vi "Example_USBCSwitch.vi"() -> ()   [LabVIEW 2021, in "BrainStem2_LabVIEW_Library.lvlib"]
uses:
  BrainStem2_LabVIEW_Library.lvlib
panel:
  out "Mux 3 Voltage":i32
  out "USB 0 CC1 Voltage":u32
  out "USB 0 CC1 Current":i32
  out "USB 0 CC2 Voltage":i32
  out "USB 0 CC1 Current":i32
  out "Mux 2 Voltage":i32
  out "USB 0 CC1 Voltage":i32
  out "USB 0 CC1 Current":i32
  out "USB 0 CC2 Voltage":i32
  out "USB 0 CC1 Current":i32
  out "Mux 1 Voltage":i32
  out "USB 0 CC1 Voltage":i32
  out "USB 0 CC1 Current":i32
  out "USB 0 CC2 Voltage":i32
  out "USB 0 CC1 Current":i32
  out "USB 0 CC2 Voltage":i32
  out "USB 0 CC1 Current":i32
  out "USB 0 CC1 Current":i32
  out "USB 0 CC1 Voltage":i32
  out "Mux 0 Voltage":i32
  out "USB 0 Voltage":i32
  out "USB 0 Current":i32
  out "USB 0 Voltage":i32
  out "USB 0 Current":i32
  out "USB 0 Voltage":i32
  out "USB 0 Current":i32
  out "USB 0 Voltage":i32
  out "USB 0 Current":i32
  # "Mux Channel 0 Values:"
  # "Mux Channel 1 Values:"
  # "Mux Channel 2 Values:"
  # "Mux Channel 3 Values:"
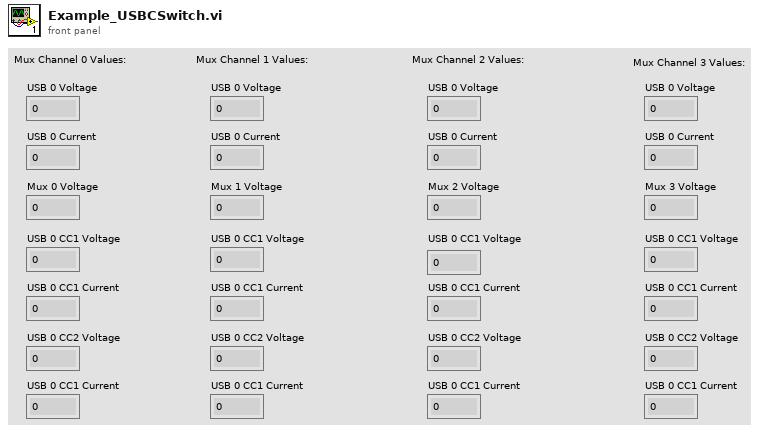
[diagram p1: front panel]
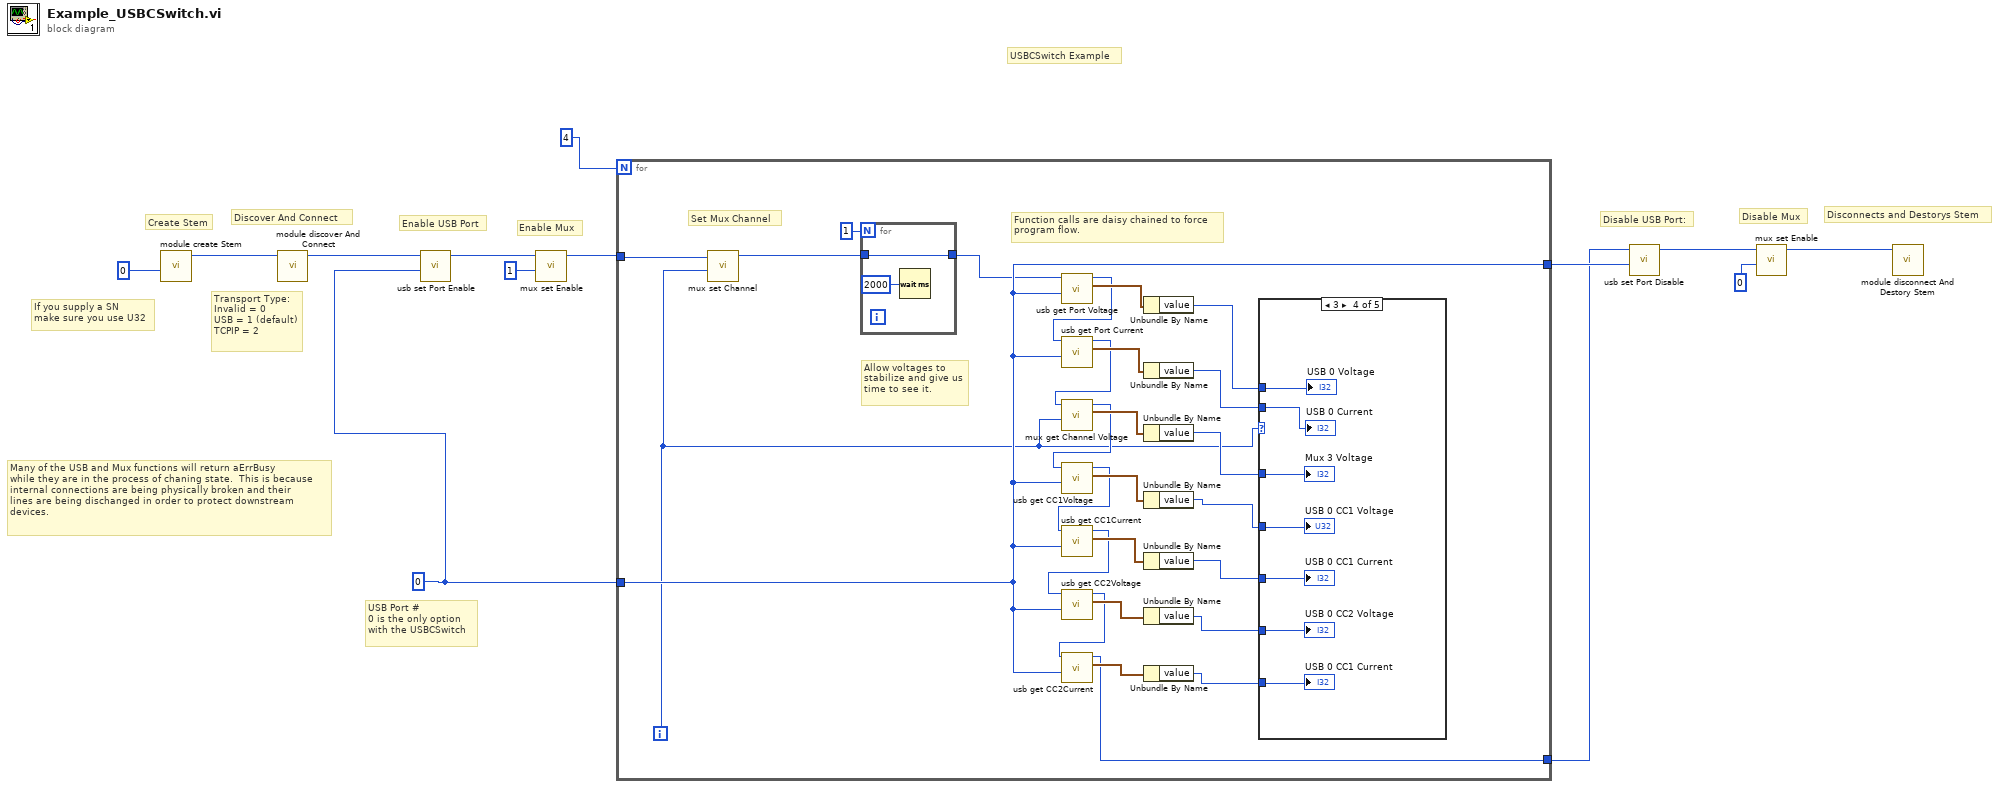
[diagram p0: block diagram]
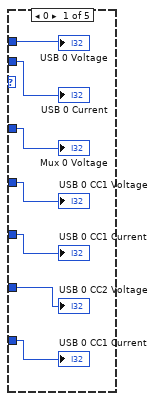
[diagram p2: hidden frame]
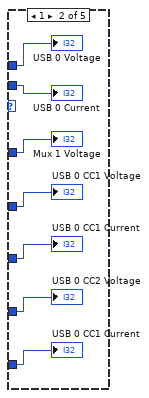
[diagram p3: hidden frame]
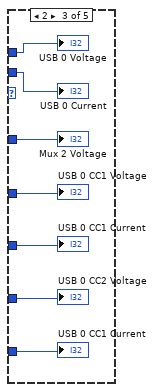
[diagram p4: hidden frame]
diagram:
  w9 = 0 ("port")
  # "Create Stem"
  # "Many of the USB and Mux functions will return aErrBusy\nwhile they are in the process of chaning state.  This is because\ninternal connections are being physically broken and their\nlines are being dischanged in order to protect downstream  \ndevices."
  # "Disable USB Port:"
  # "Discover And Connect"
  # "Disable Mux"
  # "Enable Mux"
  # "Enable USB Port"
  # "USBCSwitch Example"
  # "USB Port #\n0 is the only option\nwith the USBCSwitch"
  # "Disconnects and Destorys Stem"
  # "If you supply a SN\nmake sure you use U32"
  # "Transport Type:\nInvalid = 0\nUSB = 1 (default)\nTCPIP = 2"
  n1 = call "module create Stem.vi"("sn"=u32 0) -> ("id out"=w13:u32)  [unwired: 8 in, 2 out]
  n2 = call "module discover And Connect.vi"("id"=w13) -> ("id out"=w10:u32)  [unwired: 8 in, 2 out]
  n3 = call "usb set Port Enable.vi"("channel"=w9, "id"=w10) -> ("id out"=w8:u32)  [unwired: 7 in, 2 out]
  n4 = call "mux set Enable.vi"("index"=1 ("port"), "id"=w8) -> ("id out"=w7:u32)  [unwired: 7 in, 2 out]
  n5 = for {
    N: 4 -> [_]
    tunnel: w7 -> [w18]
    tunnel: w9 -> [w19]
    tunnel: [w20] -> w5
    tunnel: [w19] -> w6
    i -> [w17]
    # "Allow voltages to\nstabilize and give us\ntime to see it."
    # "Set Mux Channel"
    # "Function calls are daisy chained to force\nprogram flow."
    n6 = call "mux set Channel.vi"("index"=w17, "id"=w18) -> ("id out"=w15:u32)  [unwired: 7 in, 2 out]
    n7 = for {
      N: 1 -> [_]
      tunnel: [w42] -> w16
      tunnel: w15 -> [w42]
      n8 = Wait (ms)(milliseconds to wait=u32 2000) -> ()  [unwired: 1 out]
    }
    n9 = call "usb get Port Voltage.vi"("channel"=w19, "id"=w16) -> ("result out"=w40:cluster{"value":i32, "error":i32}, "id out"=w27:u32)  [unwired: 7 in, 1 out]
    n10 = call "usb get Port Current.vi"("channel"=w19, "id"=w27) -> ("result out"=w39:cluster{"value":i32, "error":i32}, "id out"=w26:u32)  [unwired: 7 in, 1 out]
    n11 = call "mux get Channel Voltage.vi"("index"=w17, "id"=w26) -> ("result out"=w38:cluster{"value":i32, "error":i32}, "id out"=w25:u32)  [unwired: 7 in, 1 out]
    n12 = call "usb get CC1Voltage.vi"("channel"=w19, "id"=w25) -> ("result out"=w37:cluster{"value":i32, "error":i32}, "id out"=w24:u32)  [unwired: 7 in, 1 out]
    n13 = call "usb get CC1Current.vi"("channel"=w19, "id"=w24) -> ("result out"=w36:cluster{"value":i32, "error":i32}, "id out"=w23:u32)  [unwired: 7 in, 1 out]
    n14 = call "usb get CC2Voltage.vi"("channel"=w19, "id"=w23) -> ("result out"=w35:cluster{"value":i32, "error":i32}, "id out"=w22:u32)  [unwired: 7 in, 1 out]
    n15 = call "usb get CC2Current.vi"("channel"=w19, "id"=w22) -> ("result out"=w34:cluster{"value":i32, "error":i32}, "id out"=w20:u32)  [unwired: 7 in, 1 out]
    n16 = Unbundle By Name(w40) -> ("value"=w33:i32)
    n17 = Unbundle By Name(w39) -> ("value"=w32:i32)
    n18 = Unbundle By Name(w38) -> ("value"=w31:i32)
    n19 = Unbundle By Name(w37) -> ("value"=w21:i32)
    n20 = Unbundle By Name(w36) -> ("value"=w30:i32)
    n21 = Unbundle By Name(w35) -> ("value"=w29:i32)
    n22 = Unbundle By Name(w34) -> ("value"=w28:i32)
    n23 = case shown="3" w17 {
      tunnel: w33 -> [w49 w56 w63 w70 _]
      tunnel: w32 -> [w48 w55 w62 w69 _]
      tunnel: w31 -> [w47 w54 w61 w68 _]
      tunnel: w21 -> [w43 w53 w60 w67 _]
      tunnel: w30 -> [w46 w52 w59 w66 _]
      tunnel: w29 -> [w45 w51 w58 w65 _]
      tunnel: w28 -> [w44 w50 w57 w64 _]
      frame 0 {
        "USB 0 Voltage" <- w49
        "USB 0 Current" <- w48
        "Mux 0 Voltage" <- w47
        "USB 0 CC1 Voltage" <- w43
        "USB 0 CC1 Current" <- w46
        "USB 0 CC2 Voltage" <- w45
        "USB 0 CC1 Current" <- w44
      }
      frame 1 {
        "Mux 1 Voltage" <- w54
        "USB 0 CC1 Voltage" <- w53
        "USB 0 CC1 Current" <- w52
        "USB 0 CC2 Voltage" <- w51
        "USB 0 CC1 Current" <- w50
        "USB 0 Voltage" <- w56
        "USB 0 Current" <- w55
      }
      frame 2 {
        "Mux 2 Voltage" <- w61
        "USB 0 CC1 Voltage" <- w60
        "USB 0 CC1 Current" <- w59
        "USB 0 CC2 Voltage" <- w58
        "USB 0 CC1 Current" <- w57
        "USB 0 Voltage" <- w63
        "USB 0 Current" <- w62
      }
      frame 3 {
        "Mux 3 Voltage" <- w68
        "USB 0 CC1 Voltage" <- w67
        "USB 0 CC1 Current" <- w66
        "USB 0 CC2 Voltage" <- w65
        "USB 0 CC1 Current" <- w64
        "USB 0 Voltage" <- w70
        "USB 0 Current" <- w69
      }
      frame 4, Default {
      }
    }
  }
  n24 = call "usb set Port Disable.vi"("channel"=w6, "id"=w5) -> ("id out"=w4:u32)  [unwired: 7 in, 2 out]
  n25 = call "mux set Enable.vi"("index"=0 ("port"), "id"=w4) -> ("id out"=w3:u32)  [unwired: 7 in, 2 out]
  n26 = call "module disconnect And Destory Stem.vi"("id"=w3) -> ()  [unwired: 8 in, 3 out]
